vi "KRH Arm Control.vi"(9 "Button Control":T1) -> (3 "Arm Angle":dbl)   [LabVIEW 2015]
uses:
  <vilib>/functionblocks/Edge Detection/One Shot Falling With Input/One Shot Falling With Input.vi
  <vilib>/functionblocks/Counter/Pulse Timer/Pulse Timer.vi
  <vilib>/functionblocks/Edge Detection/One Shot Rising with Input/One Shot Rising with Input.vi
  <vilib>/functionblocks/FB Core/FB Core.xnode
  <vilib>/functionblocks/NI_FunctionBlock Libraries.lvlib
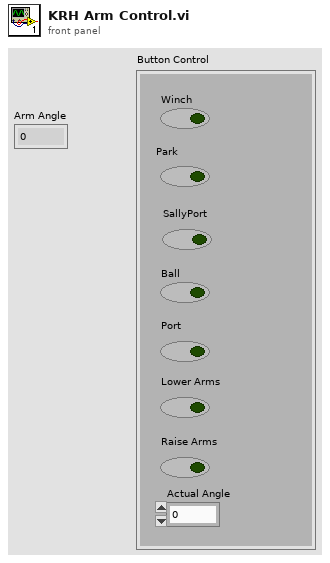
[diagram p1: front panel]
types:
  T1 = cluster{"Park":bool, "Winch":bool, "Ball":bool, "SallyPort":bool, "Port":bool, "Lower Arms":bool, "Raise Arms ":bool, "Actual Angle":dbl}
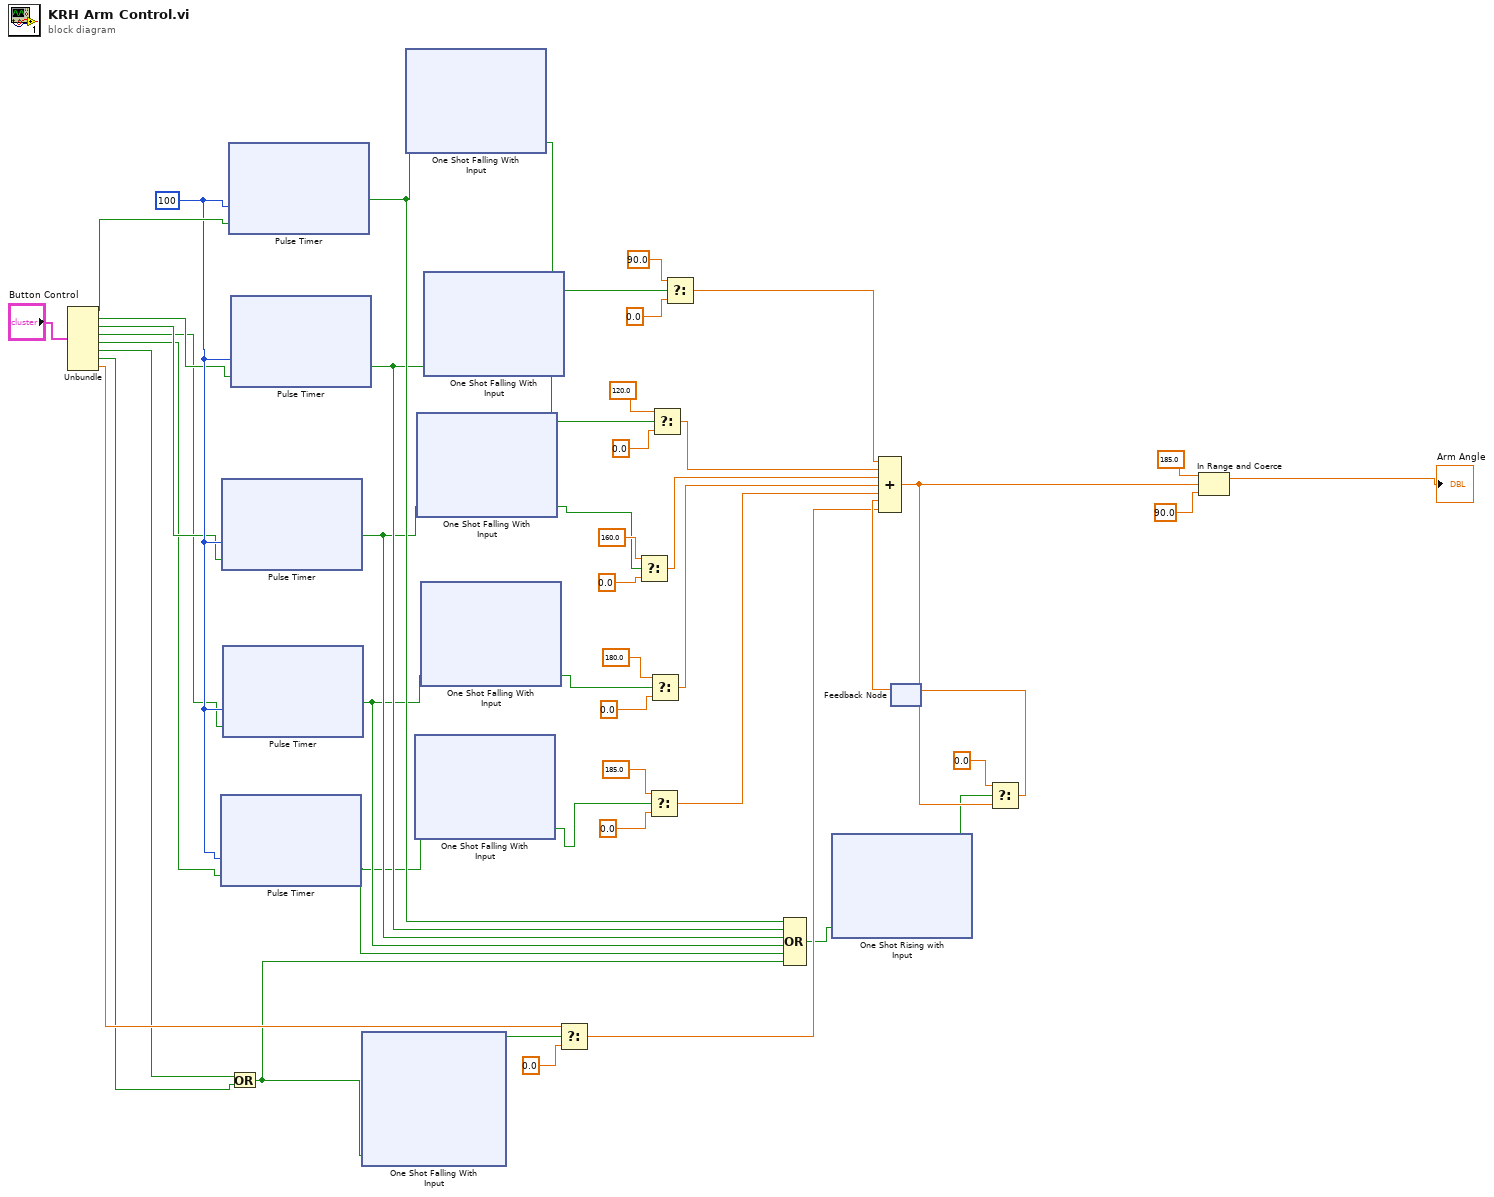
[diagram p0: block diagram]
diagram:
  w9 = 100
  n1 = Unbundle("Button Control") -> ("Park"=w20:bool, "Winch"=w8:bool, "Ball"=w7:bool, "SallyPort"=w6:bool, "Port"=w5:bool, "Lower Arms"=w23:bool, "Raise Arms"=w22:bool, "Actual Angle"=w30:dbl)
  n2 = xnode "Pulse Timer"("preset time (ms)"=w9, "input"=w5) -> ("output"=w1:bool)  [unwired: 1 in, 2 out]
  n3 = xnode "Pulse Timer"("preset time (ms)"=w9, "input"=w7) -> ("output"=w3:bool)  [unwired: 1 in, 2 out]
  n4 = xnode "Pulse Timer"("preset time (ms)"=w9, "input"=w6) -> ("output"=w2:bool)  [unwired: 1 in, 2 out]
  n5 = xnode "Pulse Timer"("preset time (ms)"=w9, "input"=w20) -> ("output"=w14:bool)  [unwired: 1 in, 2 out]
  n6 = Or(x=w23, y=w22) -> (x .or. y?=w10:bool)
  n7 = xnode "Pulse Timer"("preset time (ms)"=w9, "input"=w8) -> ("output"=w4:bool)  [unwired: 1 in, 2 out]
  n8 = xnode "One Shot Falling With Input"("input"=w10) -> ("output"=w11:bool)  [unwired: 1 in, 1 out]
  n9 = xnode "One Shot Falling With Input"("input"=w14) -> ("output"=w13:bool)  [unwired: 1 in, 1 out]
  n10 = xnode "One Shot Falling With Input"("input"=w1) -> ("output"=w17:bool)  [unwired: 1 in, 1 out]
  n11 = xnode "One Shot Falling With Input"("input"=w3) -> ("output"=w15:bool)  [unwired: 1 in, 1 out]
  n12 = xnode "One Shot Falling With Input"("input"=w2) -> ("output"=w16:bool)  [unwired: 1 in, 1 out]
  n13 = xnode "One Shot Falling With Input"("input"=w4) -> ("output"=w12:bool)  [unwired: 1 in, 1 out]
  n14 = Select(t=w30, s=w11, f=0.0) -> (s? t:f=w21:dbl)
  n15 = Select(t=160.0, s=w15, f=0.0) -> (s? t:f=w35:dbl)
  n16 = Select(t=185.0, s=w17, f=0.0) -> (s? t:f=w33:dbl)
  n17 = Select(t=180.0, s=w16, f=0.0) -> (s? t:f=w34:dbl)
  n18 = Select(t=120.0, s=w12, f=0.0) -> (s? t:f=w36:dbl)
  n19 = Select(t=90.0, s=w13, f=0.0) -> (s? t:f=w37:dbl)
  n20 = Compound Arithmetic op=OR(w14, w4, w3, w2, w1, w10) -> (w18:bool)
  n21 = xnode "One Shot Rising with Input"("input"=w18) -> ("output"=w19:bool)  [unwired: 1 in, 1 out]
  n22 = feedback #1() -> (w28:dbl)  [unwired: 1 in]
  n23 = Compound Arithmetic op=ADD(w37, w36, w35, w34, w33, w28, w21) -> (w27:dbl)
  n24 = Select(t=0.0, s=w19, f=w27) -> (s? t:f=w29:dbl)
  n25 = feedback-in #1(w29) -> ()
  n26 = In Range and Coerce(upper limit=185.0, x=w27, lower limit=90.0) -> (coerced(x)=→"Arm Angle":dbl)  [unwired: 1 out]
